vi "Construct.vi"(8 "Error in (no error)":errorcluster, 10 "Regex":string, 11 "LogFilterMessage in":refnum<class "LogFilterMessage.lvclass">) -> (0 "Error out":errorcluster, 3 "LogFilterMessage out":refnum<class "LogFilterMessage.lvclass">)   [LabVIEW 2011, in "LogFilterMessage.lvclass"]
uses:
  LogFilterMessage/LogFilterMessage.lvclass
  LogFilterMessage/LogFilterMessage.lvclass/LogFilterMessage.ctl
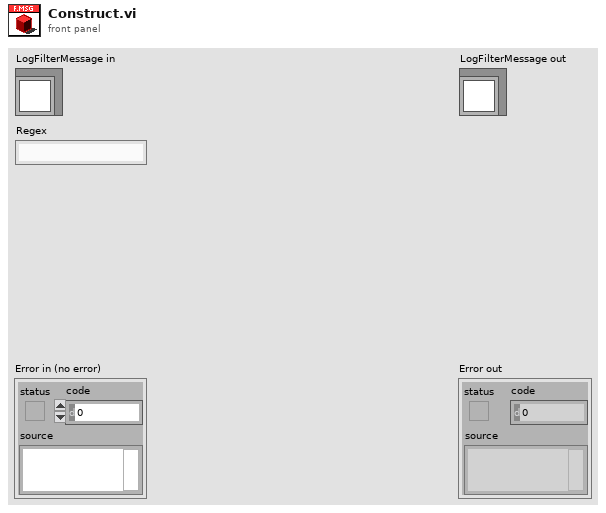
[diagram p1: front panel]
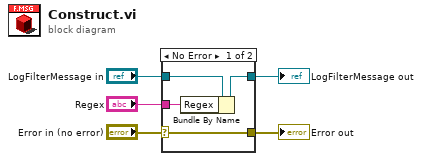
[diagram p0: block diagram]
diagram:
  n1 = case shown="No Error" "Error in (no error)" {
    selector: "Error in (no error)" -> [w9 w11]
    tunnel: [w9 w11] -> w4
    tunnel: [w6 w10] -> w2
    tunnel: "LogFilterMessage in" -> [w7 w10]
    tunnel: "Regex" -> [w8 _]
    frame No Error {
      n2 = Bundle By Name(cluster=w7, "Regex"=w8) -> (w6:refnum<class "LogFilterMessage.lvclass">)
    }
    frame Error {
    }
  }
  "Error out" <- w4
  "LogFilterMessage out" <- w2
